vi "EventInfotoEvent.vi"(2 "error in (no error)":errorcluster, 3 "JSONEventInfo":variant) -> (0 "error out":errorcluster, 1 "JSON Tree out (JSON Object)":variant)   [LabVIEW 2018]
uses:
  <vilib>/LVH/i3 JSON/JSON Generation/Create Value Files/Create Value - Object.vi
  <vilib>/LVH/i3 JSON/JSON Generation/Add Object Parameter Files/Add Object Parameter - Object.vi
  <vilib>/LVH/i3 JSON/JSON Generation/Add Object Parameter Files/Add Object Parameter - String.vi
  <vilib>/LVH/i3 JSON/i3-json.lvlib
panel:
  out "concatenated string":string
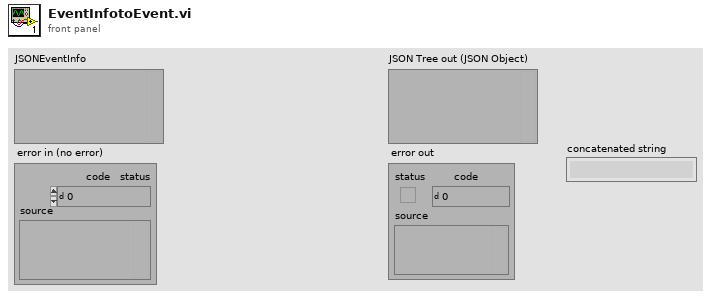
[diagram p1: front panel]
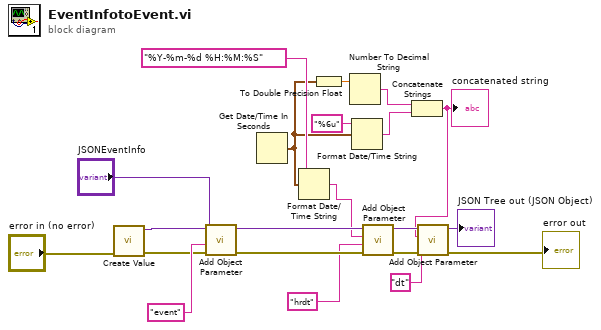
[diagram p0: block diagram]
diagram:
  n1 = call-poly <vilib>:"Create Value.vi"("error in (no error)"="error in (no error)") -> ("error out"=w3:errorcluster, "JSON Tree"=w4:variant)  [unwired: 9 in]
  n2 = call-poly <vilib>:"Add Object Parameter.vi"("error in (no error)"=w3, "Name"="event", "JSON Object"="JSONEventInfo", "JSON Tree in (JSON Object)"=w4) -> ("error out"=w20:errorcluster, "JSON Tree out (JSON Object)"=w21:variant)  [unwired: 6 in]
  n3 = Get Date/Time In Seconds() -> (seconds since 1Jan1904=w12:timestamp)
  n4 = Format Date/Time String(time format string (%c)="%Y-%m-%d %H:%M:%S", seconds (now)=w12) -> (date/time string=w16:string)  [unwired: 1 in]
  n5 = To Double Precision Float(number=w12) -> (double precision float=w11:dbl)
  n6 = Number To Decimal String(number=w11) -> (decimal integer string=w13:string)  [unwired: 1 in]
  n7 = Format Date/Time String(time format string (%c)="%6u", seconds (now)=w12) -> (date/time string=w14:string)  [unwired: 1 in]
  n8 = call-poly <vilib>:"Add Object Parameter.vi"("error in (no error)"=w20, "Name"="hrdt", "String"=w16, "JSON Tree in (JSON Object)"=w21) -> ("error out"=w9:errorcluster, "JSON Tree out (JSON Object)"=w10:variant)  [unwired: 6 in]
  n9 = Concatenate Strings(w13, w14) -> (w7:string)
  "concatenated string" <- w7
  n10 = call-poly <vilib>:"Add Object Parameter.vi"("error in (no error)"=w9, "Name"="dt", "String"=w7, "JSON Tree in (JSON Object)"=w10) -> ("error out"=→"error out":errorcluster, "JSON Tree out (JSON Object)"=→"JSON Tree out (JSON Object)":variant)  [unwired: 6 in]
